vi "Measurement_input_panel.vi"(0 "OK":T4, 2 "setup":T5, 5 "Setup filename":string) -> (11 "Setup filename out":string, 12 "Analysis Info cluster":T8[](array[typedef])=[{"Colour"=0, "Inst type"=enum."Pitot-static tube", "Inst name"="Manometer voltage", "Symbol"="U", "Code name"="", "Extra Info"="U", "Inst Array"=enum."PWA", "Extra Titles"=[], "Extra Values"=[], "U"=0.0, "u^2"=0.0, "u^3"=0.0, "u^4"=0.0, "Skew_u"=0.0, "Kurt_u"=0.0, "Sd Error in Mean"=0.0, "% u'/U"=0.0, "X"=0.0, "Y"=0.0, "Z"=0.0, "Timescale integral to 25%"=0.0, "Sd Error in Variance"=0.0, "Calib File"=path "", "Calib Constants"=[], "Output Position"=FALSE, "Full Stats"=FALSE, "Av Sampling Rate"=0.0, "Av No of Samples"=0.0, "Total Meas Time (s)"=0.0, "ADAM Ch Name"=""}, {"Colour"=0, "Inst type"=enum."Pitot-static tube", "Inst name"="Manometer voltage", "Symbol"="U", "Code name"="", "Extra Info"="U", "Inst Array"=enum."PWA", "Extra Titles"=[], "Extra Values"=[], "U"=0.0, "u^2"=0.0, "u^3"=0.0, "u^4"=0.0, "Skew_u"=0.0, "Kurt_u"=0.0, "Sd Error in Mean"=0.0, "% u'/U"=0.0, "X"=0.0, "Y"=0.0, "Z"=0.0, "Timescale integral to 25%"=0.0, "Sd Error in Variance"=0.0, "Calib File"=path "", "Calib Constants"=[], "Output Position"=FALSE, "Full Stats"=FALSE, "Av Sampling Rate"=0.0, "Av No of Samples"=0.0, "Total Meas Time (s)"=0.0, "ADAM Ch Name"=""}, {"Colour"=0, "Inst type"=enum."Pitot-static tube", "Inst name"="Manometer voltage", "Symbol"="U", "Code name"="", "Extra Info"="U", "Inst Array"=enum."PWA", "Extra Titles"=[], "Extra Values"=[], "U"=0.0, "u^2"=0.0, "u^3"=0.0, "u^4"=0.0, "Skew_u"=0.0, "Kurt_u"=0.0, "Sd Error in Mean"=0.0, "% u'/U"=0.0, "X"=0.0, "Y"=0.0, "Z"=0.0, "Timescale integral to 25%"=0.0, "Sd Error in Variance"=0.0, "Calib File"=path "", "Calib Constants"=[], "Output Position"=FALSE, "Full Stats"=FALSE, "Av Sampling Rate"=0.0, "Av No of Samples"=0.0, "Total Meas Time (s)"=0.0, "ADAM Ch Name"=""}] {"Sd Error in Variance" format="%.2f"; "Skew_u" format="%.2f"; "% u'/U" format="%.2f"; "Sd Error in Mean" format="%.2f"; "Kurt_u" format="%.2f"; "u^4" format="%.2f"; "u^3" format="%.2f"; "U" format="%.2f"; "u^2" format="%.2f"})   [LabVIEW 2012]
uses:
  Controls/Inst_type.ctl
  Controls/Analysis_info_cluster.ctl
  Controls/Instrument_Array.ctl
  Controls/LDA_Setup.ctl
  Controls/Setup.ctl
  Controls/ok_button.ctl
  Controls/Trigger_Mode.ctl
  Controls/PWA_Data.ctl
  File/Setup_Filetype.ctl
  Controls/Post_Process.ctl
  Controls/App_Global.ctl
  Controls/Ch_and_Spans.ctl
  Globals/Meas_global.vi
  Globals/Trav_pos_global.vi
  Globals/LDA_meas_global_1.vi
  Globals/Preference_global.vi
panel:
  in  "Acquisition Plug in":u16(ring) items=["ADAM_Server_Channels.vi", "DataTranslation.vi", "DataTranslation_new.vi", "DataTranslation_NM1.vi", "DataTranslation_NM2.vi", "DataTranslation_NM3.vi", "DataTranslation_old.vi", "LDA_IP.vi", "LDA_IP_DataTranslation.vi", "LDA_IP_NI-DAQmx.vi", "NI-DAQmx.vi", "Simulate_kernal.vi"]
  in  "Select Duplicate Channels":bool
  in  "PWA Data":T1
  out "Inst type":T2
  in  "Edit temp and Press":bool
  out "Abs Press (mbar)":dbl=1013.0 format="%.1f"
  out "Temp (deg C)":dbl=21.0 format="%.1f"
  in  "Trigger mode":T3
  in  "Select Plug Ins":bool
  in  "Sync Delay Time (ms)":dbl=24.0 format="%.2f"
  out "XW Present?":bool
  out "Read Setup File?":bool
  out "Setup Paths":string[](array[string])
  in  "Select Local ADAM Channels":bool
  in  "stop":bool
  out "Notes":string
  in  "Setup filename selector":u16(ring) items=["Current_Setup.xls", "Disp_Search_A.xls", "Calib_Setup.xls", "Simulate.xls", "LDA_SJ_A.xls", "LDA_only_B.xls", "LDA_only_A.xls", "NACA0015_Pressure_LDA.xls", "NACA0015_Pressure.xls", "Current_Setup.xls", "NACA0015_Pressure_LDA.xls", "NACA0015_Pressure.xls", "DT9836_test.xls", "DT_test_C.xls", "LDA_Test.xls", "SJ_Span_Test_B.xls", "DT_test_B.xls", "DT_test.xls", "NACA0015_SJ_Polar_B.xls", "NACA0015_RT_Pres_A.xls", "NACA0015_SJ_Polar_A.xls", "Calib_Setup.xls", "SJ_Indv_Test_B.xls", "NACA0015_RT_Pres_B.xls", "NACA0015_LDA_A.xls", "SJ_Indv_Test_A.xls", "SJ_Span_Test_A.xls", "NACA0015_Polar_C.xls", "SJ_Disp_A.xls", "LDA_C.xls", "SJ_Life_Test_A.xls", "LDA_D.xls", "Tare_Setup.xls", "NACA0015_Polar_B.xls", "LDA_B.xls", "LDA_A.xls", "NACA0015_Polar_A.xls", "Meas_Test.xls", "SJ_Optimisation_A.xls", "Fluidic_Switch_B.xls", "SJ_Test_Alex_A.xls", "Fluidic_Switch_A.xls", "SJ_Steel_Rig_C.xls", "SJ_Steel_Rig_B.xls", "SJ_Steel_Rig_A.xls", "HW_Calibrate_A.xls"]
  in  "Synchronise Analogue channels with LDA":bool
  in  "LDA set up":T6={"dimensions"=enum."2D", "Analogue Freq Multiplier"=0.1} {"Analogue Freq Multiplier" min=0.1 max=100.0 format="%_5g"}
  in  "LDA data":enum16{"No LDA data", "Take LDA data"}(ring)=enum."Take LDA data"
  in  "Cross wire":T7(ring)
  in  "No of Analogue inst":i32=1
  in  "Ch & spans choices":T10(array[cluster]) {"D" format="%.2f"; "Ch No" min=0; "low limit" min=-10 max=10 format="%.2f"; "high limit" min=-10 max=10 format="%.2f"}
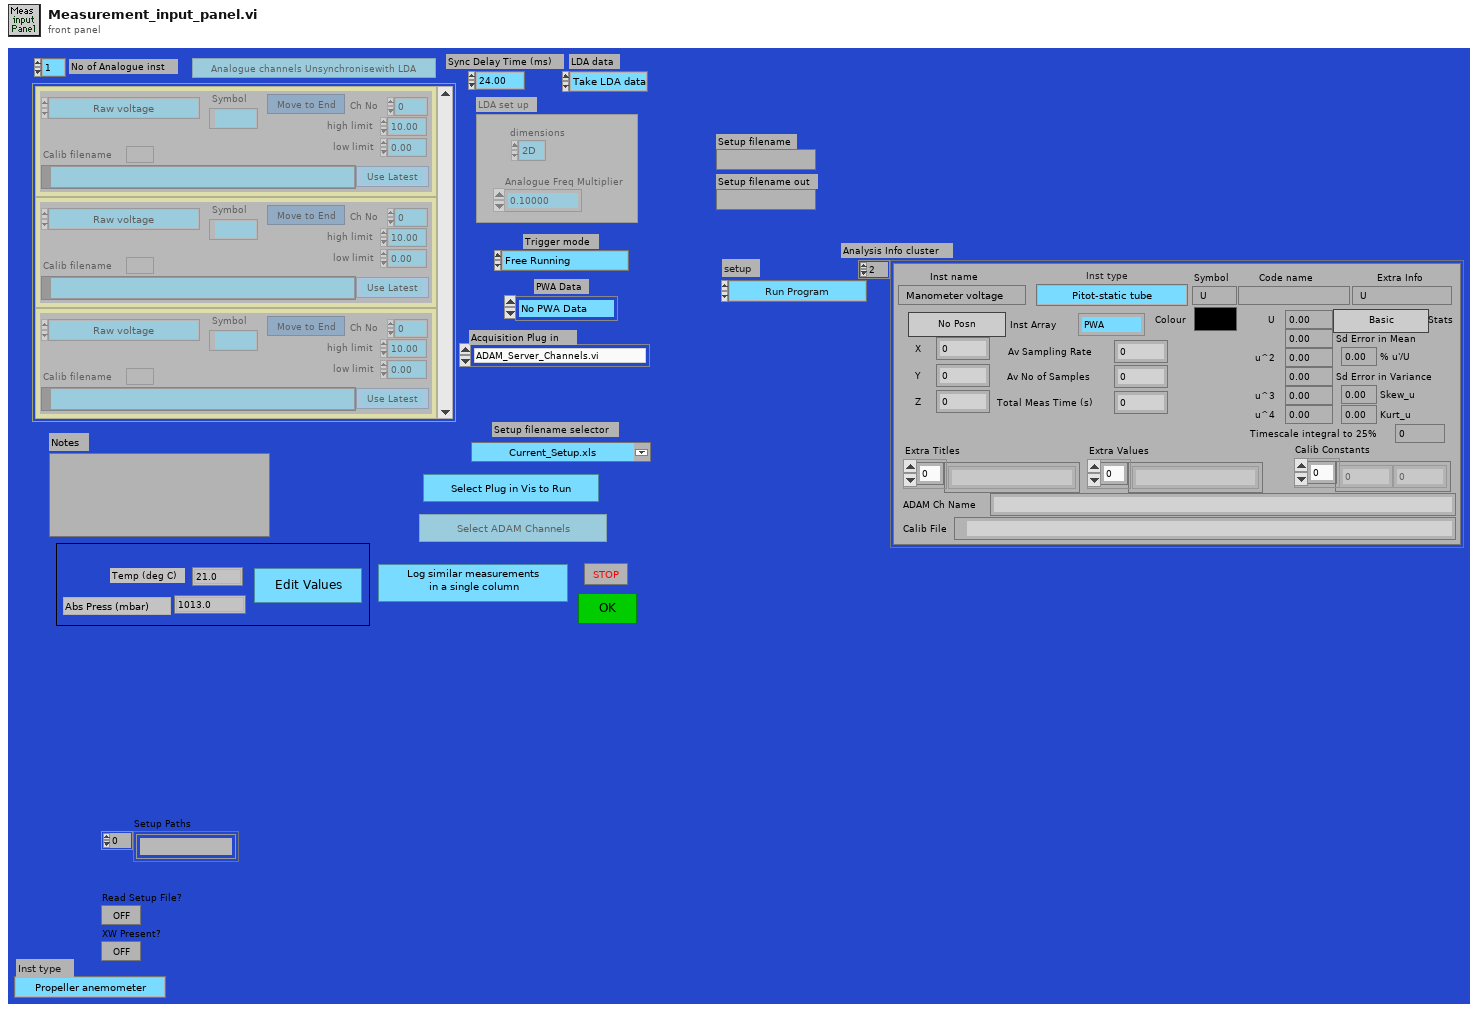
[diagram p1: front panel]
types:
  T1 = typedef "PWA_Data.ctl" = enum16{"No PWA Data", "One Ch PWA"}
  T2 = typedef "Inst_type.ctl" = enum16{"Propeller anemometer", "Raw voltage", "Pressure Transducer", "Pitot-static tube", "Preston tube", "Hot wire", "Cross wire 1", "Cross wire 2", "Generic Linear", "Generic Polynomial", "Generic BackPoly", "Fast FID", "Thermocouple", "Cold wire", "Pulsed Wire", "LDA Vel", "LDA Tran time", "LDA Arr time"}
  T3 = typedef "Trigger_Mode.ctl" = enum16{"Free Running", "Start on Trigger", "Trigger Every Block", "Trigger Every Sample"}
  T4 = typedef "ok_button.ctl" = bool
  T5 = typedef "Setup.ctl" = enum16{"Run Program", "Show Setup", "Save Current Setup", "Setup Front Panel"}
  T6 = typedef "LDA_Setup.ctl" = cluster{"dimensions":enum16{"1D", "2D"}, "Analogue Freq Multiplier":dbl}
  T7 = enum16{"2nd component as calculated", "2nd component multipled by -1"}
  T8 = typedef "Analysis_info_cluster.ctl" = cluster{"Colour":u32, "Inst type":T2, "Inst name":string, "Symbol":string, "Code name":string, "Extra Info":string, "Inst Array":T9, "Extra Titles":string[], "Extra Values":string[], "U":dbl, "u^2":dbl, "u^3":dbl, "u^4":dbl, "Skew_u":dbl, "Kurt_u":dbl, "Sd Error in Mean":dbl, "% u'/U":dbl, "X":dbl, "Y":dbl, "Z":dbl, "Timescale integral to 25%":dbl, "Sd Error in Variance":dbl, "Calib File":path, "Calib Constants":dbl[], "Output Position":bool, "Full Stats":bool, "Av Sampling Rate":dbl, "Av No of Samples":dbl, "Total Meas Time (s)":dbl, "ADAM Ch Name":string}
  T9 = typedef "Instrument_Array.ctl" = enum16{"PWA", "LDA", "Analogue"}
  T10 = cluster{"high limit":sgl, "low limit":sgl, "Ch No":i16, "Calib filename":path, "Inst type":T2, "Symbol":string, "Move channel":bool, "Use Latest":bool, "D":dbl, "Ch Name":string}[]
  T11 = typedef "Post_Process.ctl" = enum16{"Take New Data", "Post Process Raw Data File"}
  T12 = typedef "Setup_Filetype.ctl" = enum16{"Measurement Setups", "Calibration Setups", "General", "Results File Plotter Setups", "Speed Calib Tweaks"}
  T13 = typedef "App_Global.ctl" = enum16{"Read Global", "Write to Global", "Initialise Array"}
  T14 = typedef "Ch_and_Spans.ctl" = cluster{"high limit (10V)":sgl, "low limit (-10V)":sgl, "Ch No":i16, "Var name":string, "Use Latest Calib":bool}
  T15 = enum16{"Zero or one", "One", "Zero or more", "One or more"}
  T16 = typedef "Traverse_cluster.ctl" = cluster{"Start X":dbl, "Start Y":dbl, "Start Z":dbl, "End X":dbl, "End Y":dbl, "End Z":dbl, "No. of pts.":i32, "Spacing":T17, "Filename":path, "Tunnel Speed":dbl, "Averaging time (min)":dbl, "Extra Commands":string, "Specific Arguments":string, "Emission Rate (l/min)":dbl, "Trace Gas Concentration (%)":dbl, "Density Ratio":string, "Comments":string, "Row No":i32, "Row Type Selector":T18, "Completion time":string, "Row Duration (mins)":dbl, "No. of Valid pts.":i32, "Meas Setup File":string}
  T17 = typedef "Spacing.ctl" = enum16{"Linear", "Log", "Gauss", "Specified", "N/A"}
  T18 = typedef "Multi_run_mode.ctl" = enum16{"Move Traverse Only", "Set Tunnel Speed Only", "Set Source Only", "Set Measurement Conditions", "Single Measurement", "Vertical Profile", "Lateral Profile", "Longitudinal Profile", "Explore Volume", "Multi-Axis Profile", "Auto Calibrate", "Meas Fast FID Bkgnd", "Check Beam Power", "Scanning Valve Measurement", "Run VI Named:", "Set ADAM Ch", "Wait (minutes)", "Send Message", "Synchronize With:", "Fall Back to this Row", "Turn Off Row Repeating", "Blank Row", "Traverse 3D Volume"}
  T19 = cluster{"high limit (10V)":sgl, "low limit (-10V)":sgl, "Ch No":i16, "Calib filename":path, "Inst type":T2, "Symbol":string, "Move channel":bool, "Use Latest":bool, "D":dbl, "Ch Name":string}[]
  T20 = cluster{"high limit":sgl, "low limit":sgl, "Ch No":i16, "Calib filename":path, "Inst type":T2, "Symbol":string, "Move channel":bool, "Use Latest":bool, "D":dbl, "Ch Name":string}
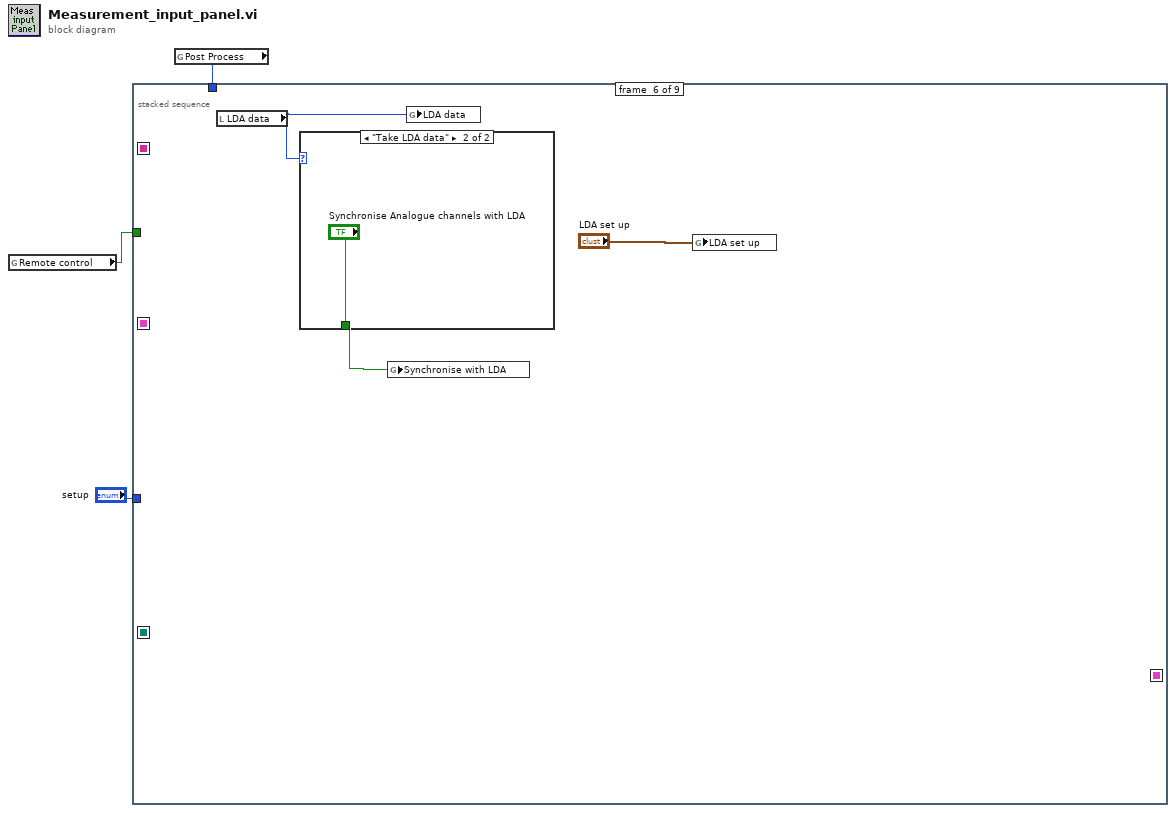
[diagram p0: block diagram]
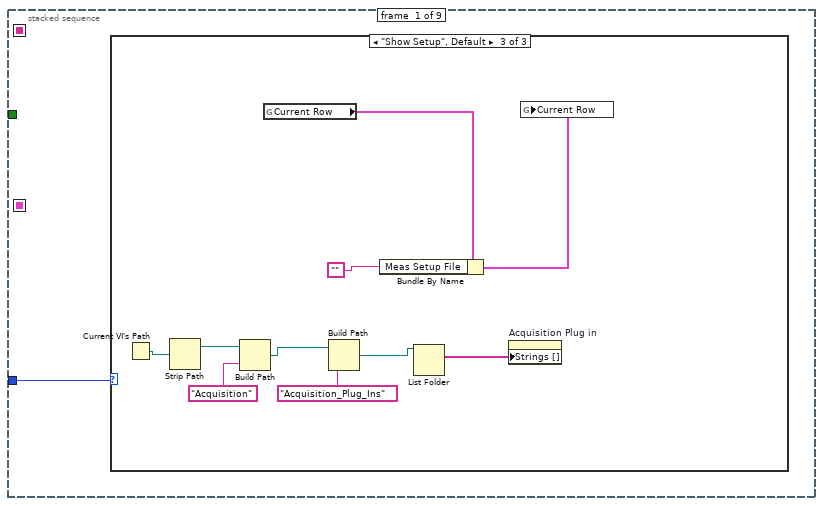
[diagram p2: hidden frame]
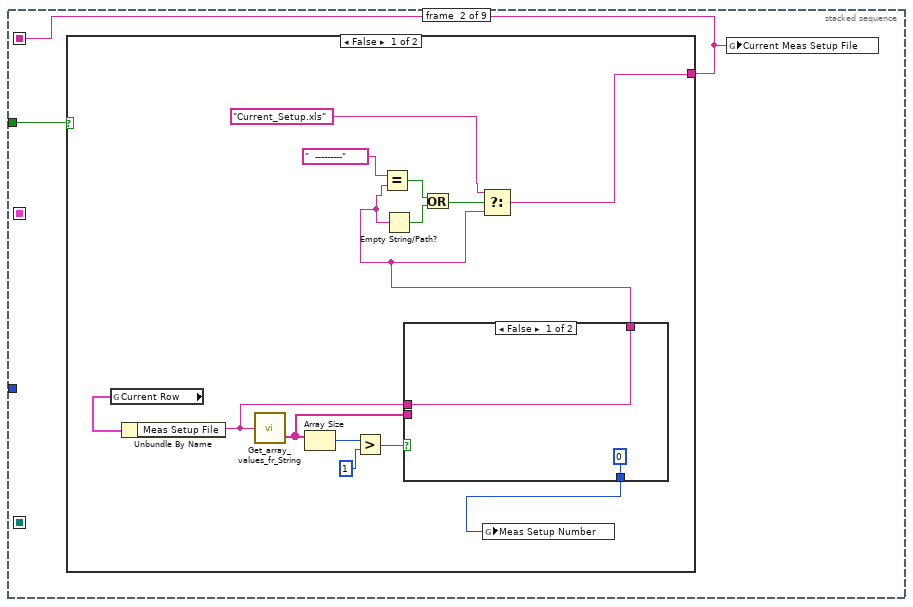
[diagram p5: hidden frame]
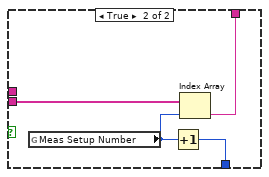
[diagram p6: hidden frame]
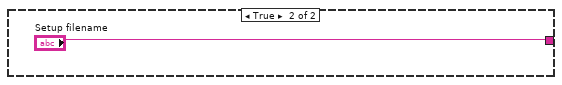
[diagram p7: hidden frame]
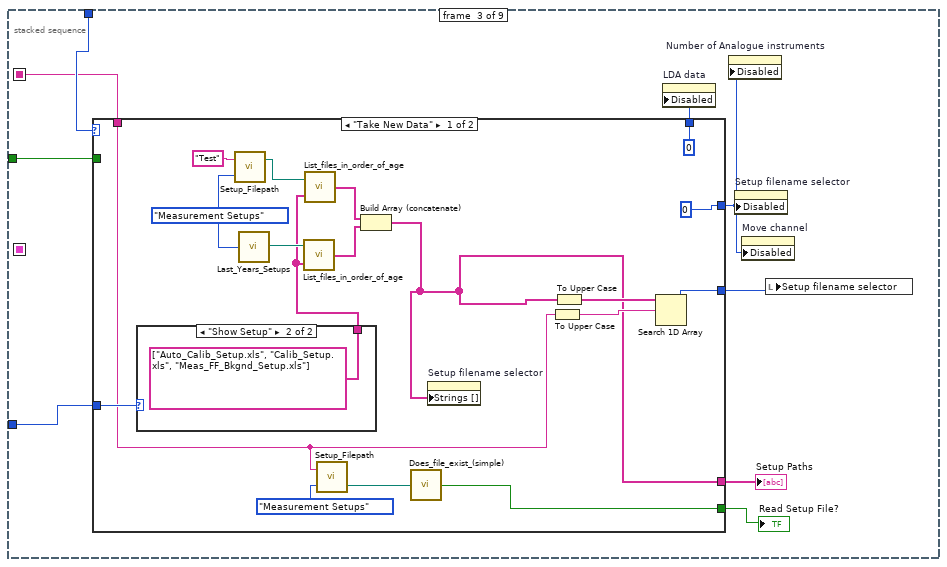
[diagram p8: hidden frame]
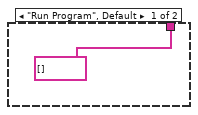
[diagram p9: hidden frame]
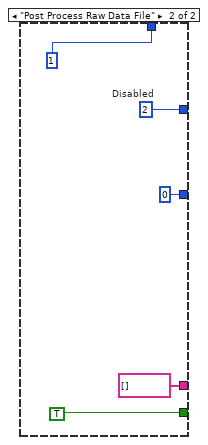
[diagram p10: hidden frame]
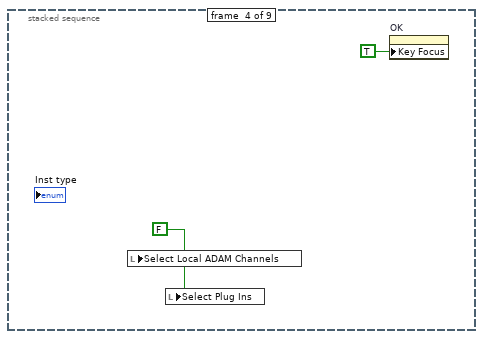
[diagram p11: hidden frame]
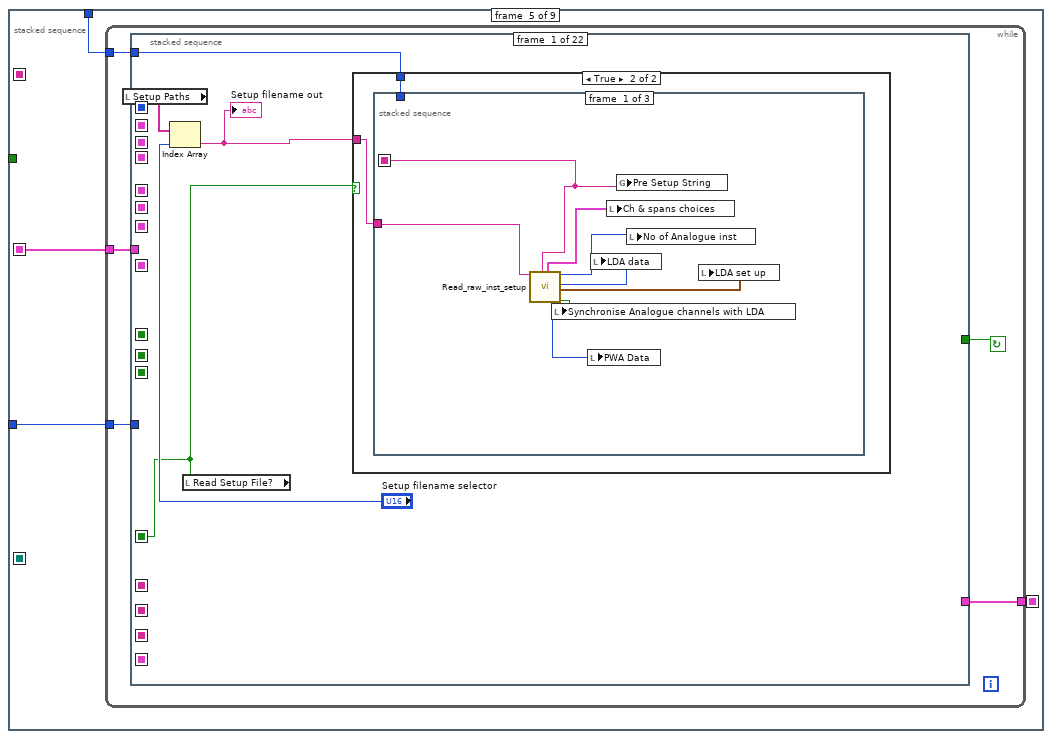
[diagram p12: hidden frame]
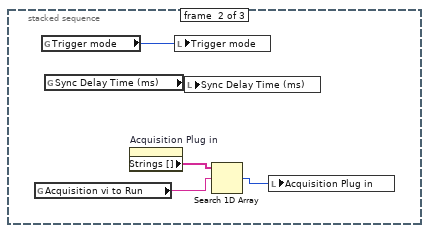
[diagram p14: hidden frame]
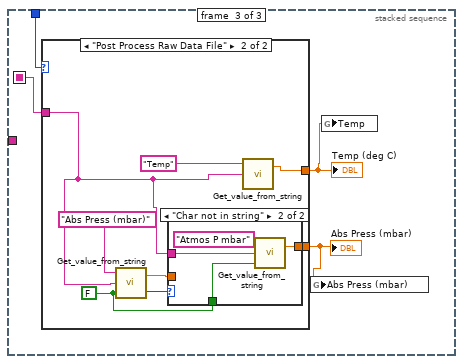
[diagram p15: hidden frame]
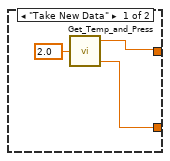
[diagram p16: hidden frame]
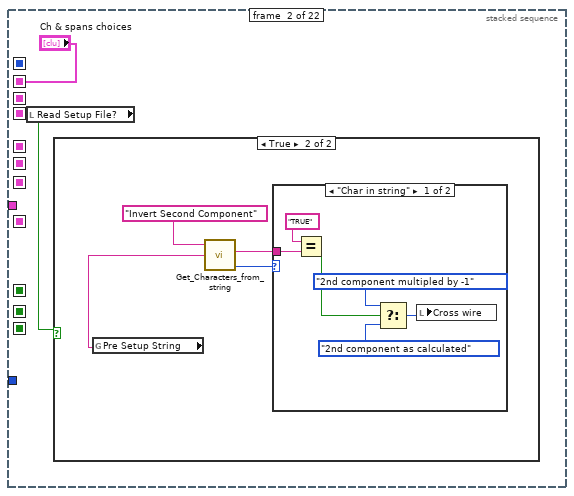
[diagram p18: hidden frame]
diagram:
  n1 = global read "Meas_global.vi" "Remote control"() -> (w1:bool)
  n2 = global read "Meas_global.vi" "Post Process"() -> (w3:T11)
  n3 = stacked-sequence {
    seq-local: [_ _ _ _ w77 _ _ _ _] -> [_ _ _ _ _ _ w693 w794 _]
    seq-local: [_ w15 _ _ _ _ _ _ _] -> [_ _ w38 _ _ _ w692 _ _]
    seq-local: [_ _ _ _ w74 _ _ _ _] -> [_ _ _ _ _ _ _ _ w846]
    seq-local: [_ _ _ _ _ _ _ w793 _] -> [_ _ _ _ _ _ _ _ w845]
    tunnel: w3 -> [_ _ w46 _ w76 _ _ w795 _]
    tunnel: "setup" -> [w4 _ w40 _ w75 _ w694 _ _]
    tunnel: w1 -> [_ w16 w39 _ _ _ _ _ _]
    frame #0 {
      n4 = case shown="\"Show Setup\", Default" w4 {
        frame "Run Program" {
        }
        frame "Setup Front Panel" {
        }
        frame "Show Setup", Default {
          n5 = Current VI's Path() -> (path=w11:path)
          n6 = Strip Path(path=w11) -> (stripped path=w10:path)  [unwired: 1 out]
          n7 = Build Path(base path=w10, name or relative path="Acquisition") -> (appended path=w7:path)
          n8 = global read "Trav_pos_global.vi" "Current Row"() -> (w14:T16)
          n9 = Build Path(base path=w7, name or relative path="Acquisition_Plug_Ins") -> (appended path=w6:path)
          n10 = Bundle By Name(cluster=w14, "Meas Setup File"="") -> (w13:T16)
          n11 = List Folder(path=w6) -> (filenames=w5:string[])  [unwired: 3 in, 3 out]
          n12 = property on="Acquisition Plug in" class="Ring (strict)"("Strings []"=w5) -> ()  [unwired: 2 in, 2 out]
          n13 = global write "Trav_pos_global.vi" "Current Row"(w13) -> ()
        }
      }
    }
    frame #1 {
      n14 = case shown="False" w16 {
        tunnel: [w29 "Setup filename"] -> w15
        frame False {
          n15 = global read "Trav_pos_global.vi" "Current Row"() -> (w25:T16)
          n16 = Unbundle By Name(w25) -> ("Meas Setup File"=w19:string)
          n17 = call "Get_array_values_fr_String.vi"("String Value"=w19) -> ("String array"=w18:string[])  [unwired: 1 out]
          n18 = Array Size(array=w18) -> (size(s)=w23:i32)
          n19 = Greater?(x=w23, y=1) -> (0:w21:bool)
          n20 = case shown="False" w21 {
            tunnel: [w32 w35] -> w20
            tunnel: w19 -> [w32 _]
            tunnel: w18 -> [_ w36]
            tunnel: [0 w33] -> w17
            frame False {
            }
            frame True {
              n21 = global read "Trav_pos_global.vi" "Meas Setup Number"() -> (w34:i32)
              n22 = Increment(x=w34) -> (x+1=w33:i32)
              n23 = Index Array(array=w36, index=w34) -> (element=w35:string)
            }
          }
          n24 = Equal?(x="  ---------" ("f"), y=w20) -> (x = y?=w28:bool)
          n25 = Empty String/Path?(string/path=w20) -> (empty?=w27:bool)
          n26 = Or(x=w28, y=w27) -> (x .or. y?=w24:bool)
          n27 = Select(t="Current_Setup.xls", s=w24, f=w20) -> (s? t:f=w29:string)
          n28 = global write "Trav_pos_global.vi" "Meas Setup Number"(w17) -> ()
        }
        frame True {
        }
      }
      n29 = global write "Trav_pos_global.vi" "Current Meas Setup File"(w15) -> ()
    }
    frame #2 {
      n30 = case shown="\"Take New Data\"" w46 {
        tunnel: [w47 string[] []] -> w42
        tunnel: [w60 TRUE ("exists")] -> w41
        tunnel: [u8 0 ("Disabled") w68] -> w43
        tunnel: [u8 0 ("Disabled") u8 1 ("Disabled")] -> w45
        tunnel: w38 -> [w56 _]
        tunnel: [w63 0 ("index of element")] -> w44
        tunnel: w40 -> [w58 _]
        tunnel: w39 -> [_ _]
        frame "Take New Data" {
          w50 = Setup_Filetype."Measurement Setups" ("Setup File Type")
          n31 = case shown="\"Show Setup\"" w58 {
            tunnel: [string[] [] ("file names") string[] ["Auto_Calib_Setup.xls", "Calib_Setup.xls", "Meas_FF_Bkgnd_Setup.xls"] ("file names")] -> w48
            frame "Run Program", Default {
            }
            frame "Show Setup" {
            }
          }
          n32 = call "Setup_Filepath.vi"("Setup File Type"=w50, "Filename in"="Test") -> ("Directory"=w51:path)  [unwired: 1 out]
          n33 = call "Last_Years_Setups.vi"("Setup File Type"=w50) -> ("Directory"=w49:path)
          n34 = call "List_files_in_order_of_age.vi"("Files to Hide"=w48, "Folder"=w49) -> ("file names"=w53:string[])
          n35 = call "List_files_in_order_of_age.vi"("Files to Hide"=w48, "Folder"=w51) -> ("file names"=w52:string[])
          n36 = call "Setup_Filepath.vi"("Setup File Type"=Setup_Filetype."Measurement Setups", "Filename in"=w56) -> ("Filename Out"=w55:path)  [unwired: 1 out]
          n37 = Build Array (concatenate)(w52, w53) -> (w47:string[])
          n38 = call "Does_file_exist_(simple).vi"("Pathname"=w55) -> ("exists?"=w60:bool)
          n39 = property on="Setup filename selector" class="Ring (strict)"("Strings []"=w47) -> ()  [unwired: 2 in, 2 out]
          n40 = To Upper Case(1:w56) -> (0:w61:string)
          n41 = To Upper Case(1:w47) -> (0:w62:string[])
          n42 = Search 1D Array(1D array=w62, element=w61) -> (index of element=w63:i32)  [unwired: 1 out]
        }
        frame "Post Process Raw Data File" {
          w68 = u8 2  # Disabled
        }
      }
      "Setup Paths" <- w42
      "Read Setup File?" <- w41
      n43 = property on="LDA data" class="Enum (strict)"("Disabled"=w45) -> ()  [unwired: 2 in, 2 out]
      n44 = property on="Number of Analogue instruments" class="DigNum (strict)"("Disabled"=w43) -> ()  [unwired: 2 in, 2 out]
      n45 = property on="Setup filename selector" class="Ring (strict)"("Disabled"=w43) -> ()  [unwired: 2 in, 2 out]
      n46 = property on="Move channel" class="Bool (strict)"("Disabled"=w43) -> ()  [unwired: 2 in, 2 out]
      n47 = local write "Setup filename selector"(w44) -> ()
    }
    frame #3 {
      w73 = FALSE ("Select Local ADAM Channels")
      n48 = local write "Select Local ADAM Channels"(w73) -> ()
      n49 = local write "Select Plug Ins"(w73) -> ()
      n50 = property on="OK" class="Bool"("Key Focus"=TRUE) -> ()  [unwired: 2 in, 2 out]
    }
    frame #4 {
      n51 = while {
        tunnel: w75 -> [w79]
        tunnel: w76 -> [w80]
        tunnel: [w82] -> w77
        tunnel: [w78] -> w74
        stop <- w81 continue-if-true
        n52 = stacked-sequence {
          seq-local: [_ _ _ _ _ _ _ _ _ w238 _ _ _ _ _ _ _ _ _ _ _ _] -> [_ _ _ _ _ _ _ _ _ _ _ w301 w346 w391 _ _ _ _ _ _ _ _]
          seq-local: [_ _ _ _ w162 _ _ _ _ _ _ _ _ _ _ _ _ _ _ _ _ _] -> [_ _ _ _ _ _ w200 _ w234 w239 _ _ _ _ _ _ _ _ _ _ _ _]
          seq-local: [_ _ _ _ _ _ w205 _ _ _ _ _ _ _ _ _ _ _ _ _ _ _] -> [_ _ _ _ _ _ _ _ _ w240 _ _ _ _ _ _ _ _ _ _ _ _]
          seq-local: [_ _ _ _ _ _ _ _ _ _ _ w303 _ _ _ _ _ _ _ _ _ _] -> [_ _ _ _ _ _ _ _ _ _ _ _ w348 _ _ _ _ _ _ _ _ w658]
          seq-local: [_ _ _ _ _ _ _ _ _ _ _ _ _ _ w424 _ _ _ _ _ _ _] -> [_ _ _ _ _ _ _ _ _ _ _ _ _ _ _ w443 _ _ _ _ _ _]
          seq-local: [_ _ _ _ _ _ _ _ _ _ _ _ _ _ _ w439 _ _ _ _ _ _] -> [_ _ _ _ _ _ _ _ _ _ _ _ _ _ _ _ w467 w533 _ _ w634 w659]
          seq-local: [_ _ _ _ _ _ _ _ _ _ _ _ w352 _ _ _ _ _ _ _ _ _] -> [_ _ _ _ _ _ _ _ _ _ _ _ _ _ w421 _ _ _ _ _ _ _]
          seq-local: [_ _ _ _ _ _ _ _ _ _ _ _ _ w395 _ _ _ _ _ _ _ _] -> [_ _ _ _ _ _ _ _ _ _ _ _ _ _ w420 _ _ _ _ _ _ _]
          seq-local: [_ _ _ _ _ _ _ _ _ _ w298 _ _ _ _ _ _ _ _ _ _ _] -> [_ _ _ _ _ _ _ _ _ _ _ w302 w349 _ _ _ _ _ _ _ _ w657]
          seq-local: [_ _ _ _ _ _ _ _ _ _ _ _ _ _ _ _ w466 _ _ _ _ _] -> [_ _ _ _ _ _ _ _ _ _ _ _ _ _ _ _ _ w536 _ _ _ _]
          seq-local: [_ _ _ _ _ _ _ _ _ _ _ _ _ _ _ _ w465 _ _ _ _ _] -> [_ _ _ _ _ _ _ _ _ _ _ _ _ _ _ _ _ w535 _ _ _ _]
          seq-local: [_ _ _ _ _ _ _ _ _ _ _ _ _ _ _ _ w464 _ _ _ _ _] -> [_ _ _ _ _ _ _ _ _ _ _ _ _ _ _ _ _ w534 _ _ _ _]
          seq-local: [_ _ _ _ _ _ _ _ _ _ _ _ _ _ _ _ _ w532 _ _ _ _] -> [_ _ _ _ _ _ _ _ _ _ _ _ _ _ _ _ _ _ _ w584 _ _]
          seq-local: [_ "Ch & spans choices" _ _ _ _ _ _ _ _ _ _ _ _ _ _ _ _ _ _ _ _] -> [_ _ _ _ w151 _ _ _ _ _ _ _ _ _ _ _ _ _ w579 _ _ _]
          seq-local: [_ _ _ _ _ _ _ _ _ _ _ _ _ _ _ _ _ w530 _ _ _ _] -> [_ _ _ _ _ _ _ _ _ _ _ _ _ _ _ _ _ _ w578 _ _ _]
          seq-local: [w83 _ _ _ _ _ _ _ _ _ _ _ _ _ _ _ _ _ _ _ _ _] -> [_ _ _ _ _ _ _ _ _ _ _ _ _ _ _ _ _ w529 _ _ _ _]
          tunnel: [_ _ _ _ _ _ _ _ _ _ _ _ _ _ _ w439 _ _ _ _ _ _] -> w82
          tunnel: [_ _ _ _ _ _ _ _ _ _ _ _ w350 _ _ _ _ _ _ _ _ _] -> w81
          tunnel: w80 -> [w85 _ _ w139 w158 _ _ _ _ _ w299 _ w347 _ w423 _ _ _ _ _ w635 _]
          tunnel: w79 -> [_ _ w135 _ _ w186 _ _ _ _ _ _ _ _ w422 _ _ _ _ w586 _ _]
          tunnel: [_ _ _ _ _ _ _ _ _ _ _ _ _ _ _ _ _ w532 _ _ _ _] -> w78
          frame #0 {
            n53 = local read "Setup Paths"() -> (w87:string[])
            n54 = Index Array(array=w87, index="Setup filename selector") -> (element=w84:string)
            "Setup filename out" <- w84
            n55 = local read "Read Setup File?"() -> (w83:bool)
            n56 = case shown="True" w83 {
              tunnel: w84 -> [_ w89]
              tunnel: w85 -> [_ w88]
              frame False {
              }
              frame True {
                n57 = stacked-sequence {
                  seq-local: [w92 _ _] -> [_ _ w105]
                  tunnel: w89 -> [w94 _ _]
                  tunnel: w88 -> [_ _ w106]
                  frame #0 {
                    n58 = call "Read_raw_inst_setup.vi"("Setup file"=w94) -> ("Setup string"=w92:string, "Ch & spans choices"=w91:T19, "PWA Data"=w90:T1, "Number of Analogue instruments"=w97:i32, "LDA data"=w96:enum16{"No LDA data", "Take LDA data"}, "LDA set up"=w93:T6, "Synchronise Analogue channels with LDA"=w95:bool)  [unwired: 12 out]
                    n59 = local write "Synchronise Analogue channels with LDA"(w95) -> ()
                    n60 = local write "PWA Data"(w90) -> ()
                    n61 = local write "LDA data"(w96) -> ()
                    n62 = local write "Ch & spans choices"(w91) -> ()
                    n63 = global write "Meas_global.vi" "Pre Setup String"(w92) -> ()
                    n64 = local write "No of Analogue inst"(w97) -> ()
                    n65 = local write "LDA set up"(w93) -> ()
                  }
                  frame #1 {
                    n66 = global read "Meas_global.vi" "Acquisition vi to Run"() -> (w99:string)
                    n67 = global read "Meas_global.vi" "Trigger mode"() -> (w101:T3)
                    n68 = global read "LDA_meas_global_1.vi" "Sync Delay Time (ms)"() -> (w102:dbl)
                    n69 = property on="Acquisition Plug in" class="Ring (strict)"() -> ("Strings []"=w100:string[])  [unwired: 2 in, 2 out]
                    n70 = local write "Trigger mode"(w101) -> ()
                    n71 = local write "Sync Delay Time (ms)"(w102) -> ()
                    n72 = Search 1D Array(1D array=w100, element=w99) -> (index of element=w98:i32)  [unwired: 1 in]
                    n73 = local write "Acquisition Plug in"(w98) -> ()
                  }
                  frame #2 {
                    n74 = case shown="\"Post Process Raw Data File\"" w106 {
                      tunnel: w105 -> [_ w112]
                      tunnel: [w107 w111] -> w103
                      tunnel: [w108 w110] -> w104
                      frame "Take New Data" {
                        n75 = call "Get_Temp_and_Press.vi"("Averaging time (mins)"=2.0) -> ("Abs Press (mbar)"=w107:dbl, "Temperature"=w108:dbl)  [unwired: 3 out]
                      }
                      frame "Post Process Raw Data File" {
                        w114 = FALSE ("Show Dialog?")
                        n76 = call "Get_value_from_string.vi"("Show Dialog?"=w114, "Input string"=w112, "Variable name"="Abs Press (mbar)") -> ("Status"=w116:enum16{"Char in string", "Char not in string"}, "Value"=w115:dbl)
                        n77 = case shown="\"Char not in string\"" w116 {
                          tunnel: [w118 w121] -> w111
                          tunnel: w115 -> [w118 _]
                          tunnel: w114 -> [_ w120]
                          tunnel: w112 -> [_ w119]
                          frame "Char in string" {
                          }
                          frame "Char not in string" {
                            n78 = call "Get_value_from_string.vi"("Show Dialog?"=w120, "Input string"=w119, "Variable name"="Atmos P mbar") -> ("Value"=w121:dbl)  [unwired: 1 out]
                          }
                        }
                        n79 = call "Get_value_from_string.vi"("Input string"=w112, "Variable name"="Temp") -> ("Value"=w110:dbl)  [unwired: 1 in, 1 out]
                      }
                    }
                    "Abs Press (mbar)" <- w103
                    "Temp (deg C)" <- w104
                    n80 = global write "Meas_global.vi" "Abs Press (mbar)"(w103) -> ()
                    n81 = global write "Meas_global.vi" "Temp"(w104) -> ()
                  }
                }
              }
            }
          }
          frame #1 {
            n82 = local read "Read Setup File?"() -> (w124:bool)
            n83 = case shown="True" w124 {
              frame False {
              }
              frame True {
                n84 = global read "Meas_global.vi" "Pre Setup String"() -> (w127:string)
                n85 = call "Get_Characters_from_string.vi"("Input string"=w127, "Variable name"="Invert Second Component") -> ("Status"=w126:enum16{"Char in string", "Char not in string"}, "Value"=w125:string)  [unwired: 1 in]
                n86 = case shown="\"Char in string\"" w126 {
                  tunnel: w125 -> [w134 _]
                  frame "Char in string" {
                    n87 = Equal?(x="TRUE", y=w134) -> (x = y?=w130:bool)
                    n88 = Select(t=T7."2nd component multipled by -1" ("Cross wire/LDA"), s=w130, f=T7."2nd component as calculated" ("Cross wire/LDA")) -> (s? t:f=w132:T7)
                    n89 = local write "Cross wire"(w132) -> ()
                  }
                  frame "Char not in string" {
                  }
                }
              }
            }
          }
          frame #2 {
            n90 = case shown="\"Show Setup\"" w135 {
              frame "Run Program", Default {
              }
              frame "Show Setup" {
                n91 = property on="Acquisition Plug in" class="Ring (strict)"() -> ("Strings []"=w138:string[])  [unwired: 2 in, 2 out]
                n92 = Index Array(array=w138, index="Acquisition Plug in") -> (element=w136:string)
                n93 = global write "Meas_global.vi" "Acquisition vi to Run"(w136) -> ()
              }
            }
          }
          frame #3 {
            n94 = case shown="True" "Edit temp and Press" {
              tunnel: w139 -> [_ w141]
              frame False {
              }
              frame True {
                n95 = case shown="\"Take New Data\"" w141 {
                  frame "Take New Data" {
                    n96 = stacked-sequence {
                      frame #0 {
                        w142 = TRUE  # Wait until done
                        n97 = call "Run_Enter_Temp.vi"("Wait until done"=w142) -> ()  [unwired: 1 out]
                      }
                      frame #1 {
                        n98 = call "Get_Temp_and_Press.vi"("Averaging time (mins)"=2.0) -> ("Abs Press (mbar)"=w143:dbl, "Temperature"=w144:dbl)  [unwired: 3 out]
                        n99 = local write "Temp (deg C)"(w144) -> ()
                        n100 = local write "Abs Press (mbar)"(w143) -> ()
                      }
                    }
                  }
                  frame "Post Process Raw Data File" {
                  }
                }
              }
            }
          }
          frame #4 {
            w154 = u8 0  # Disabled
            n101 = local read "Read Setup File?"() -> (w150:bool)
            n102 = global read "Meas_global.vi" "Acquisition vi to Run"() -> (w149:string)
            n103 = Equal?(x=w158, y=Post_Process."Take New Data" ("Post Process")) -> (x = y?=w157:bool)
            n104 = Equal?(x="ADAM_Server_Channels.vi", y=w149) -> (x = y?=w147:bool)
            n105 = And(x=w150, y=w147) -> (x .and. y?=w161:bool)
            n106 = Or(x="Select Local ADAM Channels", y=w161) -> (x .or. y?=w155:bool)
            n107 = And(x=w157, y=w155) -> (x .and. y?=w156:bool)
            n108 = case shown="True" w156 {
              tunnel: [w163 w164] -> w162
              tunnel: w151 -> [w163 w167]
              tunnel: "Select Local ADAM Channels" -> [_ w166]
              tunnel: w147 -> [_ w165]
              frame False {
              }
              frame True {
                n109 = stacked-sequence {
                  seq-local: [w168 _ _] -> [_ w178 _]
                  tunnel: w167 -> [w170 w177 _]
                  tunnel: [_ w175 _] -> w164
                  tunnel: w166 -> [w172 _ w184]
                  tunnel: w165 -> [w171 _ _]
                  frame #0 {
                    n110 = Array Size(array=w170) -> ()  [unwired: 1 out]
                    n111 = for {
                      tunnel: w170 -> [w174] mode=indexing
                      tunnel: [w173] -> w169 mode=indexing
                      n112 = Unbundle By Name(w174) -> ("Ch Name"=w173:string)
                    }
                    n113 = call "Get_local_ADAM_Chs.vi"("Local ADAM?"=w171, "Show setup"=w172, "Desired Local ADAM Channels"=w169) -> ("Choosen Channels"=w168:string[])  [unwired: 1 out]
                  }
                  frame #1 {
                    n114 = for {
                      tunnel: [w183] -> w175 mode=indexing
                      tunnel: w178 -> [w181]
                      tunnel: w177 -> [w182] mode=indexing
                      i -> [w179]
                      n115 = Index Array(array=w181, index=w179) -> (element=w180:string)
                      n116 = Bundle By Name(cluster=w182, "Ch No"=w179, "Ch Name"=w180) -> (w183:T20)
                    }
                    n117 = Array Size(array=w175) -> (size(s)=w176:i32)
                    n118 = local write "No of Analogue inst"(w176) -> ()
                  }
                  frame #2 {
                    n119 = case shown="True" w184 {
                      frame False {
                      }
                      frame True {
                        n120 = local write "Select Local ADAM Channels"(FALSE ("Select Local ADAM Channels")) -> ()
                      }
                    }
                  }
                }
              }
            }
            n121 = Select(t=w154, s=w147, f=u8 2 ("Disabled")) -> (s? t:f=w152:u8)
            n122 = property on="Ch Name" class="Str"("Visible"=w147) -> ()  [unwired: 2 in, 2 out]
            n123 = property on="Select Local ADAM Channels" class="Bool (strict)"("Disabled"=w152) -> ()  [unwired: 2 in, 2 out]
            n124 = Not(x=w147) -> (.not. x?=w146:bool)
            n125 = property on="high limit" class="DigNum (strict)"("Visible"=w146) -> ()  [unwired: 2 in, 2 out]
            n126 = property on="low limit" class="DigNum (strict)"("Visible"=w146) -> ()  [unwired: 2 in, 2 out]
            n127 = property on="Ch No" class="DigNum (strict)"("Visible"=w146) -> ()  [unwired: 2 in, 2 out]
          }
          frame #5 {
            n128 = case shown="True" "Select Plug Ins" {
              tunnel: w186 -> [_ w188]
              frame False {
              }
              frame True {
                n129 = stacked-sequence {
                  tunnel: w188 -> [w189 _]
                  frame #0 {
                    w193 = TRUE  # Show Panel?
                    n130 = global read "Meas_global.vi" "Pre Setup String"() -> (w192:string)
                    n131 = local write "Select Plug Ins"(FALSE ("Select Local ADAM Channels")) -> ()
                    n132 = call "Choose_Plug_In_to_Run.vi"("setup"=w189, "Show Panel?"=w193, "Setup String In"=w192) -> ("Setup String Out"=w191:string)  [unwired: 1 out]
                    n133 = global write "Meas_global.vi" "Pre Setup String"(w191) -> ()
                  }
                  frame #1 {
                    n134 = Current VI's Path() -> (path=w195:path)
                    n135 = call "Open_Close_Front_Panel.ph.vi"("Front Panel Window:Open"=TRUE, "VI path"=w195) -> ()  [unwired: 2 out]
                  }
                }
              }
            }
          }
          frame #6 {
            n136 = Initialize Array(0) -> (w207:i32[])  [unwired: 1 out]
            n137 = for {
              shift-right: [w214] -> w203
              shift-left: w207 -> [w215]
              tunnel: [w213] -> w201 mode=indexing
              tunnel: w200 -> [w212] mode=indexing
              tunnel: [w210] -> w199 mode=indexing
              n138 = Unbundle By Name(w212) -> ("Inst type"=w209:T2)
              n139 = case shown="\"Cross wire 1\"" w209 {
                tunnel: w215 -> [w219 w223 w225 w229]
                tunnel: [w218 w222 w225 w228] -> w214
                tunnel: [FALSE TRUE FALSE FALSE] -> w213
                frame "Propeller anemometer", Default {
                  n140 = Build Array (concatenate)(w219, 1) -> (w218:i32[])
                }
                frame "Cross wire 1" {
                  n141 = Build Array (concatenate)(w223, 2) -> (w222:i32[])
                }
                frame "Cross wire 2" {
                }
                frame "LDA Vel" {
                  n142 = Build Array (concatenate)(w229, 1) -> (w228:i32[])
                }
              }
              n143 = Equal?(x=w209, y=Inst_type."Preston tube" ("Inst type")) -> (x = y?=w210:bool)
            }
            n144 = Build Array (concatenate)(w203, 1) -> (w202:i32[])
            n145 = Array Subset(array=w202, length="No of Analogue inst") -> (w206:i32[])  [unwired: 1 in]
            n146 = Add Array Elements(numeric array=w206) -> (sum=w205:i32)
            n147 = Or Array Elements(Boolean array=w201) -> (logical OR=→"XW Present?":bool)
            n148 = Or Array Elements(Boolean array=w199) -> (logical OR=w197:bool)
            n149 = property on="D" class="DigNum (strict)"("Visible"=w197) -> ()  [unwired: 2 in, 2 out]
          }
          frame #7 {
            "Notes" <- ""
          }
          frame #8 {
            n150 = Array Size(array=w234) -> (size(s)=w233:i32)
            n151 = Not Equal To 0?(x=w233) -> (x != 0?=w232:bool)
            n152 = case shown="True" w232 {
              tunnel: [enum16{"No Analogue data", "Take Analogue data"}."No Analogue data" ("Analogue data") enum16{"No Analogue data", "Take Analogue data"}."Take Analogue data" ("Analogue data")] -> w231
              frame False {
              }
              frame True {
              }
            }
            n153 = global write "Meas_global.vi" "Analogue data"(w231) -> ()
          }
          frame #9 {
            n154 = Index Array(array=w239, index=0) -> (element=w244:T20)
            n155 = Initialize Array(w244) -> (w242:T10)  [unwired: 1 out]
            n156 = Build Array (concatenate)(w239, w244) -> (w243:T10)
            n157 = for {
              N: w240 -> [_]
              tunnel: w243 -> [w252] mode=indexing
              shift-right: [w253] -> w238
              shift-left: w242 -> [w247]
              tunnel: Inst_type."Cross wire 2" ("Inst type") -> [w245]
              shift-right: [w251] -> _
              shift-left: _ -> [w250]
              tunnel: w243 -> [w249]
              n158 = Unbundle By Name(w252) -> ("Inst type"=w251:T2)
              n159 = Array Size(array=w247) -> (size(s)=w246:i32)
              n160 = Increment(x=w246) -> (x+1=w248:i32)
              n161 = case shown="\"Cross wire 1\"" w251 {
                tunnel: [w262 w283 w295] -> w253
                tunnel: w247 -> [w263 w285 w297]
                tunnel: w252 -> [w259 w286 w296]
                tunnel: w245 -> [w261 w290 _]
                tunnel: w250 -> [_ w289 _]
                tunnel: w249 -> [w266 _ _]
                tunnel: w248 -> [w265 _ _]
                frame "Cross wire 1" {
                  n162 = Index Array(array=w266, index=w265) -> (element=w260:T20)
                  n163 = Unbundle By Name(w260) -> ("Inst type"=w264:T2, "high limit"=w257:sgl, "low limit"=w256:sgl, "Ch No"=w255:i16, "Symbol"=w254:string)
                  n164 = Unbundle By Name(w259) -> ("Calib filename"=w258:path)
                  n165 = case shown="\"Generic Linear\", Default" w264 {
                    tunnel: w263 -> [w276 w282]
                    tunnel: [w275 w281] -> w262
                    tunnel: w261 -> [w268 w277]
                    tunnel: w258 -> [w274 w280]
                    tunnel: w259 -> [w272 w278]
                    tunnel: w260 -> [_ _]
                    tunnel: w257 -> [w271 _]
                    tunnel: w256 -> [w270 _]
                    tunnel: w255 -> [w269 _]
                    tunnel: w254 -> [w267 _]
                    frame "Cross wire 2" {
                      n166 = Bundle By Name(cluster=w272, "Calib filename"=w274, "Inst type"=w268, "high limit"=w271, "low limit"=w270, "Ch No"=w269, "Symbol"=w267) -> (w273:T20)
                      n167 = Build Array (concatenate)(w276, w272, w273) -> (w275:T10)
                    }
                    frame "Generic Linear", Default {
                      n168 = Bundle By Name(cluster=w278, "Calib filename"=w280, "Inst type"=w277) -> (w279:T20)
                      n169 = Build Array (concatenate)(w282, w278, w279) -> (w281:T10)
                    }
                  }
                }
                frame "Cross wire 2" {
                  n170 = Decrement(x=w290) -> (x-1=w288:T2)
                  n171 = Equal?(x=w288, y=w289) -> (x = y?=w287:bool)
                  n172 = Bundle By Name(cluster=w286, "Inst type"=w288) -> (w284:T20)
                  n173 = case shown="False" w287 {
                    tunnel: w286 -> [_ _]
                    tunnel: w285 -> [w293 w294]
                    tunnel: w284 -> [w292 _]
                    tunnel: [w291 w294] -> w283
                    frame False {
                      n174 = Build Array (concatenate)(w293, w292) -> (w291:T10)
                    }
                    frame True {
                    }
                  }
                }
                frame "Generic Linear", Default {
                  n175 = Build Array (concatenate)(w297, w296) -> (w295:T10)
                }
              }
            }
          }
          frame #10 {
            n176 = Equal?(x=w299, y=Post_Process."Take New Data" ("Post Process")) -> (x = y?=w298:bool)
          }
          frame #11 {
            n177 = case shown="True" "OK" {
              tunnel: w301 -> [_ w318]
              tunnel: [FALSE w317] -> w303
              tunnel: w302 -> [_ w306]
              frame False {
              }
              frame True {
                n178 = for {
                  tunnel: w318 -> [w330] mode=indexing
                  tunnel: [w328] -> w312 mode=indexing
                  tunnel: [w324] -> w316 mode=indexing
                  n179 = Unbundle By Name(w330) -> ("high limit"=w333:sgl, "low limit"=w332:sgl, "Ch No"=w329:i16, "Inst type"=w327:T2, "Symbol"=w326:string)
                  n180 = Number To Decimal String(number=w327) -> (decimal integer string=w325:string)  [unwired: 1 out]
                  n181 = Concatenate Strings(w325, w326) -> (w324:string)
                  n182 = Greater Or Equal?(x=w333, y=w332) -> (x >= y?=w331:bool)
                  n183 = case shown="\"Propeller anemometer\", Default" w327 {
                    tunnel: w331 -> [w336 _ _ _]
                    tunnel: w329 -> [w335 _ _ _]
                    tunnel: [w334 TRUE TRUE TRUE] -> w328
                    frame "Propeller anemometer", Default {
                      n184 = case shown="True" w336 {
                        tunnel: w335 -> [w339 _]
                        tunnel: [FALSE TRUE] -> w334
                        frame False {
                          n185 = Number To Decimal String(number=w339) -> (decimal integer string=w338:string)  [unwired: 1 out]
                          n186 = Concatenate Strings("Error in input limits for Channel No ", w338) -> (w340:string)
                          n187 = One Button Dialog(message=w340) -> ()  [unwired: 2 out]
                        }
                        frame True {
                        }
                      }
                    }
                    frame "LDA Vel" {
                    }
                    frame "LDA Tran time" {
                    }
                    frame "LDA Arr time" {
                    }
                  }
                }
                n188 = call "Analyse_string_array.vi"("String array"=w316) -> ("Frequency"=w315:i32[])  [unwired: 2 out]
                n189 = global read "Meas_global.vi" "Remote control"() -> (w307:bool)
                n190 = Greater?(x=w315, y=1) -> (0:w313:bool[])
                n191 = Or Array Elements(Boolean array=w313) -> (logical OR=w309:bool)
                n192 = Compound Arithmetic op=AND(invert w307, w309, w306) -> (w308:bool)
                n193 = case shown="True" w308 {
                  tunnel: [TRUE FALSE] -> w311
                  frame False {
                  }
                  frame True {
                    n194 = Current VI's Path() -> (path=w321:path)
                    n195 = call "Open_Close_Front_Panel.ph.vi"("Front Panel Window:Open"=TRUE, "VI path"=w321) -> ()  [unwired: 2 out]
                    n196 = One Button Dialog(message="Non Unique symbol names") -> ()  [unwired: 2 out]
                  }
                }
                n197 = Build Array (concatenate)(w312, w311) -> (w310:bool[])
                n198 = And Array Elements(Boolean array=w310) -> (logical AND=w317:bool)
              }
            }
          }
          frame #12 {
            n199 = And(x=w349, y=w348) -> (x .and. y?=w351:bool)
            n200 = case shown="True" w351 {
              tunnel: w346 -> [_ w359]
              tunnel: [FALSE w358] -> w352
              tunnel: [w353 w357] -> w350
              tunnel: w348 -> [w354 _]
              tunnel: w347 -> [_ _]
              frame False {
                n201 = Not(x=w354) -> (.not. x?=w353:bool)
              }
              frame True {
                n202 = for {
                  shift-right: [w378] -> _
                  shift-left: i16[] [] -> [w377]
                  tunnel: w359 -> [w374] mode=indexing
                  tunnel: [w365] -> w360 mode=indexing
                  shift-right: [w373] -> _
                  shift-left: path[] [] -> [w372]
                  n203 = Unbundle By Name(w374) -> ("Ch No"=w375:i16)
                  n204 = Unbundle By Name(w374) -> ("Inst type"=w371:T2, "Calib filename"=w368:path)
                  n205 = Search 1D Array(1D array=w377, element=w375) -> (index of element=w376:i32)  [unwired: 1 out]
                  n206 = Build Array (concatenate)(w377, w375) -> (w378:i16[])
                  n207 = Equal?(x=Inst_type."Fast FID" ("Inst type"), y=w371) -> (x = y?=w364:bool)
                  n208 = case shown="0, Default" w376 {
                    tunnel: w375 -> [w389 _]
                    tunnel: [w385 FALSE ("true")] -> w367
                    frame 0, Default {
                      n209 = Format Into String(format string="The Ch No %d appears more than once", w389) -> (resulting string=w387:string)  [unwired: 2 in, 1 out]
                      n210 = One Button Dialog(message=w387, button name ("OK")="Ok") -> (true=w385:bool)
                    }
                    frame -1 {
                    }
                  }
                  n211 = Search 1D Array(1D array=w372, element=w368) -> (index of element=w369:i32)  [unwired: 1 out]
                  n212 = Greater Or Equal To 0?(x=w369) -> (x >= 0?=w363:bool)
                  n213 = And(x=w364, y=w363) -> (x .and. y?=w362:bool)
                  n214 = case shown="True" w362 {
                    tunnel: [w380 FALSE ("true")] -> w366
                    tunnel: w368 -> [w379 _]
                    frame True {
                      n215 = Format Into String(format string="Calibration file %s is used more than once.", w379) -> (resulting string=w382:string)  [unwired: 2 in, 1 out]
                      n216 = One Button Dialog(message=w382, button name ("OK")="Ok") -> (true=w380:bool)
                    }
                    frame False {
                    }
                  }
                  n217 = Build Array (concatenate)(w372, w368) -> (w373:path[])
                  n218 = Or(x=w367, y=w366) -> (x .or. y?=w365:bool)
                }
                n219 = Or Array Elements(Boolean array=w360) -> (logical OR=w357:bool)
                n220 = Not(x=w357) -> (.not. x?=w358:bool)
              }
            }
          }
          frame #13 {
            n221 = call "Current_Calib_Filenames.vi"("Mode"=App_Global."Read Global") -> ("Calib Filename Out"=w392:path[], "Channel Numbers Out"=w393:i16[])  [unwired: 2 in, 1 out]
            n222 = for {
              tunnel: w391 -> [w406] mode=indexing
              tunnel: w393 -> [w408]
              tunnel: w392 -> [w407]
              tunnel: [w405] -> w395 mode=indexing
              w403 = Inst_type."Cross wire 2"  # Inst type
              n223 = Unbundle By Name(w406) -> ("Inst type"=w398:T2, "Ch No"=w400:i16, "Use Latest"=w401:bool, "Inst type"=w404:T2)
              n224 = Not Equal?(x=w404, y=w403) -> (x != y?=w402:bool)
              n225 = Compound Arithmetic op=AND(w401, w402) -> (w399:bool)
              n226 = Not Equal?(x=Inst_type."Raw voltage" ("Inst type"), y=w398) -> (x != y?=w396:bool)
              n227 = case shown="True" w399 {
                tunnel: w408 -> [_ w419]
                tunnel: w400 -> [_ w418]
                tunnel: w407 -> [_ w416]
                tunnel: w406 -> [w409 w415]
                tunnel: [w409 w414] -> w405
                tunnel: w396 -> [_ w411]
                frame False {
                }
                frame True {
                  n228 = Search 1D Array(1D array=w419, element=w418) -> (index of element=w417:i32)  [unwired: 1 out]
                  n229 = Index Array(array=w416, index=w417) -> (element=w412:path)
                  n230 = Select(t=w412, s=w411, f=path "") -> (s? t:f=w413:path)
                  n231 = Bundle By Name(cluster=w415, "Calib filename"=w413) -> (w414:T20)
                }
              }
            }
          }
          frame #14 {
            n232 = case shown="True" w421 {
              tunnel: w420 -> [w425 w428]
              tunnel: [w425 w427] -> w424
              tunnel: w423 -> [_ _]
              tunnel: w422 -> [_ w426]
              frame False {
              }
              frame True {
                n233 = case shown="\"Run Program\", Default" w426 {
                  tunnel: w428 -> [w430 w438]
                  tunnel: [w429 w438] -> w427
                  frame "Run Program", Default {
                    n234 = for {
                      tunnel: w430 -> [w431] mode=indexing
                      tunnel: [w432] -> w429 mode=indexing
                      n235 = Unbundle By Name(w431) -> ("Calib filename"=w437:path, "Use Latest"=w436:bool, "Ch No"=w435:i16, "Inst type"=w434:T2)
                      n236 = call "Find_calibration_file.vi"("Inst type"=w434, "Ch No"=w435, "Use Latest Calib"=w436, "filename"=w437) -> ("filename out"=w433:path)
                      n237 = Bundle By Name(cluster=w431, "Calib filename"=w433) -> (w432:T20)
                    }
                  }
                  frame "Setup Front Panel" {
                  }
                }
              }
            }
          }
          frame #15 {
            w441 = 0 ("Index")
            n238 = Index Array(array=w443, index=w441) -> (element=w442:T20)
            n239 = Initialize Array(w442, w441) -> (w440:T10)
            n240 = for {
              shift-right: [w451] -> w445
              shift-left: w440 -> [w450]
              shift-right: [w452] -> w446
              shift-left: w440 -> [w454]
              tunnel: w443 -> [w453] mode=indexing
              n241 = Unbundle By Name(w453) -> ("Move channel"=w455:bool)
              n242 = case shown="True" w455 {
                tunnel: w454 -> [w457 w463]
                tunnel: w453 -> [w459 w462]
                tunnel: [w458 w463] -> w452
                tunnel: [w456 w461] -> w451
                tunnel: w450 -> [w456 w460]
                frame False {
                  n243 = Build Array (concatenate)(w457, w459) -> (w458:T10)
                }
                frame True {
                  n244 = Build Array (concatenate)(w460, w462) -> (w461:T10)
                }
              }
            }
            n245 = Build Array (concatenate)(w446, w445) -> (w444:T10)
            n246 = for {
              tunnel: w444 -> [w449] mode=indexing
              tunnel: [w447] -> w439 mode=indexing
              n247 = Bundle By Name(cluster=w449, "Move channel"=FALSE) -> (w447:T20)
            }
          }
          frame #16 {
            n248 = for {
              shift-right: [w473] -> _
              shift-left: string[] [] -> [w474]
              tunnel: [w476] -> w465 mode=indexing
              tunnel: [w470] -> w466 mode=indexing
              tunnel: w467 -> [w472] mode=indexing
              tunnel: [w469] -> w464 mode=indexing
              n249 = Unbundle By Name(w472) -> ("Inst type"=w475:T2)
              n250 = case shown="\"Propeller anemometer\"" w475 {
                tunnel: [w483 w487 w490 w494 w498 w502 w506 "XW" w513 w518 w521 w525] -> w470
                tunnel: ["U" "P" "U" "U" "tau" "U" "U" "W" "U" "C" "T" "T"] -> w477
                tunnel: w474 -> [w484 w488 w492 w496 w500 w504 w508 w510 w515 w519 w523 w527]
                tunnel: [w482 w486 w491 w495 w499 w503 w507 w510 w514 w517 w522 w526] -> w473
                frame "Propeller anemometer" {
                  w483 = "Prop"
                  n251 = Build Array (concatenate)(w484, w483) -> (w482:string[])
                }
                frame "Pressure Transducer" {
                  w487 = "Mano"
                  n252 = Build Array (concatenate)(w488, w487) -> (w486:string[])
                }
                frame "Raw voltage" {
                  w490 = "RV"
                  n253 = Build Array (concatenate)(w492, w490) -> (w491:string[])
                }
                frame "Pitot-static tube" {
                  w494 = "Pitot"
                  n254 = Build Array (concatenate)(w496, w494) -> (w495:string[])
                }
                frame "Preston tube" {
                  w498 = "Preston"
                  n255 = Build Array (concatenate)(w500, w498) -> (w499:string[])
                }
                frame "Hot wire" {
                  w502 = "HW"
                  n256 = Build Array (concatenate)(w504, w502) -> (w503:string[])
                }
                frame "Cross wire 1" {
                  w506 = "XW"
                  n257 = Build Array (concatenate)(w508, w506) -> (w507:string[])
                }
                frame "Cross wire 2" {
                }
                frame "Generic Linear", Default {
                  w513 = "Gen"
                  n258 = Build Array (concatenate)(w515, w513) -> (w514:string[])
                }
                frame "Fast FID" {
                  w518 = "FF"
                  n259 = Build Array (concatenate)(w519, w518) -> (w517:string[])
                }
                frame "Thermocouple" {
                  w521 = "T"
                  n260 = Build Array (concatenate)(w523, w521) -> (w522:string[])
                }
                frame "Cold wire" {
                  w525 = "CW"
                  n261 = Build Array (concatenate)(w527, w525) -> (w526:string[])
                }
              }
              n262 = call "Analyse_string_array.vi"("String array"=w473) -> ("Unique strings"=w481:string[], "Frequency"=w479:i32[])  [unwired: 1 out]
              n263 = Search 1D Array(1D array=w481, element=w470) -> (index of element=w480:i32)  [unwired: 1 out]
              n264 = Index Array(array=w479, index=w480) -> (element=w471:i32)
              n265 = Number To Decimal String(number=w471) -> (decimal integer string=w469:string)  [unwired: 1 out]
              n266 = Concatenate Strings(w469, w470, ":", w477) -> (w476:string)
            }
          }
          frame #17 {
            w539 = T8 {"Colour"=0, "Inst type"=enum."Pitot-static tube", "Inst name"="Manometer voltage", "Symbol"="U", "Code name"="", "Extra Info"="U", "Inst Array"=enum."PWA", "Extra Titles"=[], "Extra Values"=[], "U"=0.0, "u^2"=0.0, "u^3"=0.0, "u^4"=0.0, "Skew_u"=0.0, "Kurt_u"=0.0, "Sd Error in Mean"=0.0, "% u'/U"=0.0, "X"=0.0, "Y"=0.0, "Z"=0.0, "Timescale integral to 25%"=0.0, "Sd Error in Variance"=0.0, "Calib File"=path "", "Calib Constants"=[], "Output Position"=FALSE, "Full Stats"=FALSE, "Av Sampling Rate"=0.0, "Av No of Samples"=0.0, "Total Meas Time (s)"=0.0, "ADAM Ch Name"=""}  # Analysis info cluster
            n267 = property on="Ch Name" class="Str"() -> ("Visible"=w540:bool)  [unwired: 2 in, 2 out]
            n268 = global read "Meas_global.vi" "Pre Setup String"() -> (w531:string)
            n269 = for {
              tunnel: [w571] -> w538 mode=indexing
              tunnel: w533 -> [w547] mode=indexing
              tunnel: w536 -> [w562] mode=indexing
              tunnel: T14 {"high limit (10V)"=10.0, "low limit (-10V)"=-10.0, "Ch No"=0, "Var name"="", "Use Latest Calib"=FALSE} ("Ch and Spans") -> [w568]
              tunnel: [w567] -> w532 mode=indexing
              tunnel: w535 -> [w550] mode=indexing
              tunnel: w539 -> [w565]
              tunnel: w534 -> [w559] mode=indexing
              tunnel: w540 -> [w542]
              tunnel: w531 -> [w551]
              tunnel: [w546] -> w530 mode=indexing
              tunnel: w529 -> [w541]
              n270 = Unbundle By Name(w547) -> ("Use Latest"=w563:bool, "high limit"=w570:sgl, "low limit"=w569:sgl, "Ch No"=w564:i16, "Inst type"=w557:T2, "Symbol"=w556:string, "D"=w555:dbl, "Ch Name"=w543:string)
              n271 = Empty String/Path?(string/path=w556) -> (empty?=w560:bool)
              n272 = Concatenate Strings(w550, "_ADAM_Ch_Name" ("string")) -> (w548:string)
              n273 = call "Get_Characters_from_string.vi"("Input string"=w551, "Variable name"=w548) -> ("Value"=w545:string)  [unwired: 1 in, 1 out]
              n274 = Select(t=w559, s=w560, f=w556) -> (s? t:f=w558:string)
              n275 = Format Into String(format string="%s (%s)" ("Format String"), w562, w558) -> (resulting string=w553:string)  [unwired: 2 in, 1 out]
              n276 = Select(t=w543, s=w542, f=w553) -> (s? t:f=w552:string)
              n277 = Bundle By Name(cluster=w568, "Use Latest Calib"=w563, "high limit (10V)"=w570, "low limit (-10V)"=w569, "Ch No"=w564, "Var name"=w552) -> (w571:T14)
              n278 = Select(t=w545, s=w541, f=w543) -> (s? t:f=w544:string)
              n279 = case shown="\"Propeller anemometer\", Default" w557 {
                tunnel: [w574 w577] -> w566
                tunnel: w564 -> [w572 _]
                tunnel: w555 -> [_ w575]
                frame "Propeller anemometer", Default {
                  n280 = Format Into String(format string="Ch %d" ("Format String"), w572) -> (resulting string=w574:string)  [unwired: 2 in, 1 out]
                }
                frame "Preston tube" {
                  n281 = Format Into String(format string="D = %.2f" ("Format String"), w575) -> (resulting string=w577:string)  [unwired: 2 in, 1 out]
                }
              }
              n282 = Bundle By Name(cluster=w547, "Ch Name"=w544) -> (w546:T20)
              n283 = Bundle By Name(cluster=w565, "Extra Info"=w566, "Inst type"=w557, "Inst name"=w553, "Symbol"=w558, "Code name"=w550, "Inst Array"=Instrument_Array."Analogue", "ADAM Ch Name"=w544) -> (w567:T8)
            }
            n284 = global write "Meas_global.vi" "Ch & spans"(w538) -> ()
          }
          frame #18 {
            n285 = Not Equal?(x=w579, y=w578) -> (x != y?=w580:bool)
            n286 = case shown="True" w580 {
              tunnel: w578 -> [_ w581]
              frame False {
              }
              frame True {
                n287 = local write "Ch & spans choices"(w581) -> ()
              }
            }
          }
          frame #19 {
            n288 = global read "Meas_global.vi" "Duplicate channels"() -> (w583:i32[])
            n289 = case shown="True" "Select Duplicate Channels" {
              tunnel: w586 -> [_ _]
              tunnel: w584 -> [w594 w617]
              tunnel: w583 -> [w588 w610]
              tunnel: [w587 w609] -> w582
              frame False {
                n290 = for {
                  tunnel: w594 -> [w608] mode=indexing
                  tunnel: [w607] -> w595 mode=indexing
                  n291 = Unbundle By Name(w608) -> ("Inst type"=w607:T2)
                }
                n292 = for {
                  tunnel: w588 -> [w604] mode=indexing
                  tunnel: w595 -> [w606]
                  tunnel: [w605] -> w599 mode=indexing
                  tunnel: [w604] -> w596 mode=indexing
                  n293 = Index Array(array=w606, index=w604) -> (element=w605:T2)
                }
                n294 = Array Size(array=w594) -> (size(s)=w597:i32)
                n295 = Array Max & Min(array=w599) -> (max value=w600:T2, min value=w601:T2)  [unwired: 2 out]
                n296 = Array Max & Min(array=w596) -> (max index (indices)=w598:i32)  [unwired: 3 out]
                n297 = Array Size(array=w588) -> (size(s)=w593:i32)
                n298 = Equal?(x=w600, y=w601) -> (x = y?=w603:bool)
                n299 = Greater?(x=w593, y=1) -> (0:w590:bool)
                n300 = Greater?(x=w597, y=w598) -> (0:w602:bool)
                n301 = Compound Arithmetic op=AND(w590, w603, w602) -> (w589:bool)
                n302 = Select(t=w588, s=w589, f=i32[] [] ("32bit integer")) -> (s? t:f=w587:i32[])
              }
              frame True {
                n303 = for {
                  tunnel: w617 -> [w624] mode=indexing
                  shift-right: [w619] -> w613
                  shift-left: string[] [] -> [w620]
                  tunnel: w610 -> [w622]
                  tunnel: [w618] -> w612 mode=indexing
                  i -> [w623]
                  n304 = Unbundle By Name(w624) -> ("Inst name"=w618:string)
                  n305 = Search 1D Array(1D array=w622, element=w623) -> (index of element=w621:i32)  [unwired: 1 out]
                  n306 = case shown="0, Default" w621 {
                    tunnel: w620 -> [w627 w628]
                    tunnel: w618 -> [w626 _]
                    tunnel: [w625 w628] -> w619
                    frame 0, Default {
                      n307 = Build Array (concatenate)(w627, w626) -> (w625:string[])
                    }
                    frame -1 {
                    }
                  }
                }
                n308 = call "Select_Strings.vi"("Available Ch names"=w612, "Message"="Please select similar instruments whose results columns will be combined", "Selector mode"=T15."Zero or more", "Desired Ch names (in)"=w613) -> ("Ch Indicies Choosen"=w609:i32[])  [unwired: 4 out]
                n309 = local write "Select Duplicate Channels"(FALSE ("Select Local ADAM Channels")) -> ()
              }
            }
            n310 = global write "Meas_global.vi" "Duplicate channels"(w582) -> ()
          }
          frame #20 {
            n311 = local read "XW Present?"() -> (w631:bool)
            n312 = property on="Cross wire/LDA" class="Enum (strict)"("Visible"=w631) -> ()  [unwired: 2 in, 2 out]
            n313 = case shown="\"Take LDA data\"" "LDA data" {
              tunnel: [w640 w643] -> w633
              tunnel: w634 -> [_ w641]
              tunnel: w635 -> [_ _]
              tunnel: [w640 w642] -> w630
              frame "No LDA data" {
                w639 = FALSE  # Synchronise Analogue channels with LDA
                w640 = u8 2  # Disabled
                n314 = local write "Synchronise Analogue channels with LDA"(w639) -> ()
              }
              frame "Take LDA data" {
                n315 = stacked-sequence {
                  tunnel: [w644 _] -> w643
                  tunnel: [_ w646] -> w642
                  tunnel: w641 -> [_ w647]
                  frame #0 {
                    w644 = u8 0  # Disabled
                  }
                  frame #1 {
                    n316 = Array Size(array=w647) -> (size(s)=w648:i32)
                    n317 = Not Equal To 0?(x=w648) -> (x != 0?=w645:bool)
                    n318 = case shown="False" w645 {
                      tunnel: w645 -> [w650 _]
                      tunnel: [w649 w651] -> w646
                      frame False {
                        w649 = u8 2  # Disabled
                        n319 = local write "Synchronise Analogue channels with LDA"(w650) -> ()
                      }
                      frame True {
                        w651 = u8 0  # Disabled
                      }
                    }
                  }
                }
              }
            }
            n320 = case shown="True" w631 {
              tunnel: [w637 "Cross wire"] -> w629
              frame False {
                w637 = T7."2nd component as calculated"  # Cross wire/LDA
              }
              frame True {
              }
            }
            n321 = global write "Meas_global.vi" "Cross wire + or -ve"(w629) -> ()
            n322 = Wait (ms)(milliseconds to wait=u32 100) -> ()  [unwired: 1 out]
            n323 = property on="Synchronise Analogue channels with LDA" class="Bool (strict)"("Disabled"=w630) -> ()  [unwired: 2 in, 2 out]
            n324 = property on="LDA set up" class="Clust (strict)"("Disabled"=w633) -> ()  [unwired: 2 in, 2 out]
          }
          frame #21 {
            n325 = And(x=w657, y=w658) -> (x .and. y?=w656:bool)
            n326 = local read "Synchronise Analogue channels with LDA"() -> (w655:bool)
            n327 = while {
              shift-left: _ -> [w684]
              shift-right: [w685] -> w652
              tunnel: [w686] -> w654
              stop <- FALSE continue-if-true
              n328 = local read "Setup filename selector"() -> (w685:u16)
              n329 = Not Equal?(x=w685, y=w684) -> (x != y?=w686:bool)
            }
            n330 = case shown="True" w655 {
              tunnel: w659 -> [_ w670]
              tunnel: w656 -> [_ w669]
              frame False {
              }
              frame True {
                n331 = case shown="True" w669 {
                  tunnel: w670 -> [_ w673]
                  frame False {
                  }
                  frame True {
                    n332 = for {
                      tunnel: w673 -> [w682] mode=indexing
                      tunnel: [w675] -> w672 mode=indexing
                      n333 = Unbundle By Name(w682) -> ("Inst type"=w681:T2, "Symbol"=w679:string)
                      n334 = Equal?(x=w679, y="Sync") -> (x = y?=w677:bool)
                      n335 = Equal?(x=Inst_type."Raw voltage" ("Inst type"), y=w681) -> (x = y?=w676:bool)
                      n336 = And(x=w676, y=w677) -> (x .and. y?=w675:bool)
                    }
                    n337 = Or Array Elements(Boolean array=w672) -> (logical OR=w671:bool)
                    n338 = case shown="False" w671 {
                      frame False {
                        n339 = One Button Dialog(message="To Perform LDA Sync you must provide a Raw voltage channel having the symbol \"Sync\"") -> ()  [unwired: 2 out]
                      }
                      frame True {
                      }
                    }
                  }
                }
              }
            }
            n340 = case shown="True" w654 {
              tunnel: [FALSE ("exists?") w668] -> w653
              tunnel: w652 -> [_ w666]
              frame False {
              }
              frame True {
                n341 = local read "Setup Paths"() -> (w667:string[])
                n342 = Index Array(array=w667, index=w666) -> (element=w664:string)
                n343 = call "Setup_Filepath.vi"("Setup File Type"=Setup_Filetype."Measurement Setups", "Filename in"=w664) -> ("Filename Out"=w663:path)  [unwired: 1 out]
                n344 = call "Does_file_exist_(simple).vi"("Pathname"=w663) -> ("exists?"=w668:bool)
              }
            }
            n345 = local write "Read Setup File?"(w653) -> ()
            n346 = Current VI's Path() -> (path=w660:path)
            n347 = call "Close_Panel_and_Abort.vi"("Vi path"=w660, "stop"="stop") -> ()  [unwired: 1 out]
          }
        }
      }
    }
    frame #5 {
      n348 = local read "LDA data"() -> (w689:enum16{"No LDA data", "Take LDA data"})
      n349 = case shown="\"Take LDA data\"" w689 {
        tunnel: [FALSE ("Synchronise Analogue channels with LDA") "Synchronise Analogue channels with LDA"] -> w688
        frame "No LDA data" {
        }
        frame "Take LDA data" {
        }
      }
      n350 = global write "Meas_global.vi" "Synchronise with LDA"(w688) -> ()
      n351 = global write "Meas_global.vi" "LDA data"(w689) -> ()
      n352 = global write "Meas_global.vi" "LDA set up"("LDA set up") -> ()
    }
    frame #6 {
      n353 = stacked-sequence {
        seq-local: [_ w729 _ _] -> [_ _ _ w787]
        seq-local: [_ _ w755 _] -> [_ _ _ w786]
        seq-local: [w697 _ _ _] -> [_ _ _ w774]
        tunnel: w694 -> [w696 _ _ w778]
        tunnel: w693 -> [_ _ _ w777]
        tunnel: w692 -> [w695 _ _ _]
        frame #0 {
          n354 = local read "PWA Data"() -> (w698:T1)
          n355 = case shown="\"One Ch PWA\"" w698 {
            tunnel: ["" w707] -> w697
            tunnel: w696 -> [_ w706]
            tunnel: w695 -> [_ w702]
            frame "No PWA Data" {
            }
            frame "One Ch PWA" {
              n356 = Not Equal?(x="Calib_Setup.xls", y=w702) -> (x != y?=w701:bool)
              n357 = case shown="\"Setup Front Panel\"" w706 {
                tunnel: [w711 w714 w717 w720] -> w705
                tunnel: [w710 w713 w716 w719] -> w704
                tunnel: [w709 w712 w715 w718] -> w700
                tunnel: w701 -> [w709 w712 w715 _]
                frame "Show Setup" {
                  w711 = TRUE  # Show Panel?
                  w710 = T4 FALSE  # OK
                }
                frame "Run Program" {
                  w714 = FALSE  # Show Panel?
                  w713 = T4 TRUE  # OK
                }
                frame "Save Current Setup" {
                  w717 = FALSE  # Show Panel?
                  w716 = T4 TRUE  # OK
                }
                frame "Setup Front Panel" {
                  w718 = FALSE  # Check Calib file?
                  w720 = FALSE  # Show Panel?
                  w719 = T4 TRUE  # OK
                }
              }
              n358 = global read "Meas_global.vi" "Pre Setup String"() -> (w708:string)
              n359 = call "PWA_Setup_Panel.vi"("Show Panel?"=w705, "Check Calib file?"=w700, "OK"=w704, "Incoming Setup String"=w708) -> ("Outgoing Setup String"=w707:string)  [unwired: 3 out]
            }
          }
        }
        frame #1 {
          n360 = local read "LDA set up"() -> (w734:T6)
          n361 = global read "Meas_global.vi" "Duplicate channels"() -> (w733:i32[])
          n362 = Unbundle By Name(w734) -> ("dimensions"=w726:enum16{"1D", "2D"}, "Analogue Freq Multiplier"=w724:dbl)
          n363 = case shown="\"2D\"" w726 {
            tunnel: ["1D" "2D"] -> w728
            frame "1D" {
            }
            frame "2D" {
            }
          }
          n364 = for {
            shift-right: [w737] -> w731
            shift-left: "" -> [w740]
            tunnel: w733 -> [w741] mode=indexing
            n365 = Number To Decimal String(number=w741) -> (decimal integer string=w739:string)  [unwired: 1 out]
            n366 = Concatenate Strings(w740, w739, "; ") -> (w737:string)
          }
          n367 = call "Characters_to_string.vi"("Characters to write"=w728, "Label for characters"="LDA Dimensions") -> ("Output string"=w727:string)
          n368 = call "Value_to_string.vi"("Value"=w724, "Label for value"="LDA Analog Freq Multiplier") -> ("Output string"=w721:string)  [unwired: 1 in]
          n369 = call "Characters_to_string.vi"("Characters to write"=w731, "Label for characters"="Log_Similar_Measurements_in_the _same_column") -> ("Output string"=w722:string)
          n370 = Concatenate Strings(w727, w721, w722) -> (w729:string)
        }
        frame #2 {
          n371 = global write "Meas_global.vi" "Trigger mode"("Trigger mode") -> ()
          n372 = local read "Cross wire"() -> (w758:T7)
          n373 = global read "Preference_global.vi" "Rig Setup"() -> (w744:string)
          n374 = Match Pattern(string=w744, regular expression="-") -> (before substring=w743:string)  [unwired: 4 out]
          n375 = case shown="\"Free Running\"" "Trigger mode" {
            tunnel: ["Free Running" "Trigger Every Block" "Trigger Every Sample" "Start on Trigger"] -> w753
            frame "Free Running" {
            }
            frame "Trigger Every Block" {
            }
            frame "Trigger Every Sample" {
            }
            frame "Start on Trigger" {
            }
          }
          n376 = property on="PWA Data" class="Enum (strict)"() -> ("Strings []"=w749:string[])  [unwired: 2 in, 2 out]
          n377 = global write "Meas_global.vi" "PWA Data"("PWA Data") -> ()
          n378 = Equal?(x=T7."2nd component multipled by -1" ("Cross wire/LDA"), y=w758) -> (x = y?=w757:bool)
          n379 = case shown="\"EnFlo_Tunnel\"" w743 {
            tunnel: ["" w765] -> w742
            frame "False", Default {
            }
            frame "EnFlo_Tunnel" {
              n380 = call "Characters_to_string.vi"("Characters to write"="FALSE", "Label for characters"="Show_all_EnFlo_Tunnel_Columns") -> ("Output string"=w765:string)
            }
          }
          n381 = Index Array(array=w749, index="PWA Data") -> (element=w748:string)
          n382 = Select(t="TRUE", s=w757, f="FALSE") -> (s? t:f=w760:string)
          n383 = call "Characters_to_string.vi"("Characters to write"=w748, "Label for characters"="Pulsed_Wire_Data" ("Variable name")) -> ("Output string"=w747:string)
          n384 = call "Characters_to_string.vi"("Characters to write"=w760, "Label for characters"="Invert Second Component") -> ("Output string"=w756:string)
          n385 = call "Characters_to_string.vi"("Characters to write"=w753, "Label for characters"="Trigger mode") -> ("Output string"=w751:string)
          n386 = Concatenate Strings(w751, w747, w756, w742) -> (w755:string)
        }
        frame #3 {
          w779 = FALSE  # Show Panel?
          n387 = for {
            tunnel: w777 -> [w792] mode=indexing
            tunnel: [w791] -> w773 mode=indexing
            n388 = Unbundle By Name(w792) -> ("Ch Name"=w791:string)
          }
          n389 = global read "Meas_global.vi" "Pre Setup String"() -> (w780:string)
          n390 = call "Choose_Plug_In_to_Run.vi"("setup"=w778, "Show Panel?"=w779, "Setup String In"=w780) -> ("Setup String Out"=w781:string)  [unwired: 1 out]
          n391 = Array To Spreadsheet String(array=w773, 3:"%s" ("format string")) -> (spreadsheet string=w775:string)  [unwired: 1 out]
          n392 = call "Add_label_to_string.vi"("String to write"=w775, "File Label"="Local ADAM Channels") -> ("Output string"=w788:string)
          n393 = call "Date_and_Time_to_string.vi"() -> ("Date and time (spreadsheet)"=w783:string)
          n394 = global read "Meas_global.vi" "New Setup String"() -> (w782:string)
          n395 = call "Value_to_string.vi"("Value"="Sync Delay Time (ms)", "Label for value"="Sync Delay Time (ms)" ("Label for characters")) -> ("Output string"=w776:string)  [unwired: 1 in]
          n396 = Concatenate Strings(w782, w774, w781, w783, w787, w786, w788, w776) -> (w790:string)
          n397 = global write "Meas_global.vi" "New Setup String"(w790) -> ()
          n398 = global write "LDA_meas_global_1.vi" "Sync Delay Time (ms)"("Sync Delay Time (ms)") -> ()
        }
      }
    }
    frame #7 {
      n399 = case shown="\"Post Process Raw Data File\"" w795 {
        tunnel: w794 -> [w802 w837]
        tunnel: [w796 w831] -> w793
        frame "Take New Data" {
          n400 = for {
            tunnel: w802 -> [w813] mode=indexing
            shift-right: [w809] -> w799
            shift-left: i16[] [] -> [w811]
            shift-right: [w807] -> w798
            shift-left: path[] [] -> [w808]
            tunnel: [w804] -> w796 mode=indexing
            n401 = Unbundle By Name(w813) -> ("Use Latest"=w806:bool, "Inst type"=w812:T2, "Ch No"=w810:i16, "Calib filename"=w805:path)
            n402 = call "Current_Filepath.vi"("Filename in"=w805, "Data Type"="Calibrations") -> ("Filename Out"=w804:path)  [unwired: 1 out]
            n403 = case shown="\"Propeller anemometer\", Default" w812 {
              tunnel: w811 -> [w820 w830]
              tunnel: w810 -> [w819 _]
              tunnel: [w818 w830] -> w809
              tunnel: w808 -> [w817 w829]
              tunnel: w805 -> [w816 _]
              tunnel: [w815 w829] -> w807
              tunnel: w806 -> [w814 _]
              frame "Propeller anemometer", Default {
                n404 = case shown="False" w814 {
                  tunnel: w820 -> [w826 w828]
                  tunnel: w819 -> [w825 _]
                  tunnel: [w824 w828] -> w818
                  tunnel: w817 -> [w823 w827]
                  tunnel: w816 -> [w822 _]
                  tunnel: [w821 w827] -> w815
                  frame False {
                    n405 = Build Array (concatenate)(w826, w825) -> (w824:i16[])
                    n406 = Build Array (concatenate)(w823, w822) -> (w821:path[])
                  }
                  frame True {
                  }
                }
              }
              frame "Raw voltage" {
              }
            }
          }
          n407 = call "Current_Calib_Filenames.vi"("Calib Filename"=w798, "Channel Numbers"=w799, "Mode"=App_Global."Write to Global") -> ()  [unwired: 3 out]
        }
        frame "Post Process Raw Data File" {
          n408 = for {
            tunnel: w837 -> [w843] mode=indexing
            tunnel: [w842] -> w831 mode=indexing
            n409 = Unbundle By Name(w843) -> ("Calib filename"=w842:path)
          }
          n410 = global read "Meas_global.vi" "Pre Setup String"() -> (w836:string)
          n411 = call "Get_Characters_from_string.vi"("Input string"=w836, "Variable name"="Skip_Block_Numbers_(eg 1;2;5;12)") -> ("Status"=w834:enum16{"Char in string", "Char not in string"}, "Value"=w833:string)  [unwired: 1 in]
          n412 = case shown="\"Char in string\"" w834 {
            tunnel: w833 -> [w840 _]
            tunnel: [w838 i32[] []] -> w832
            frame "Char in string" {
              n413 = call "Get_array_values_fr_String.vi"("String Value"=w840) -> ("Numeric Array"=w839:dbl[])  [unwired: 1 out]
              n414 = To Long Integer(number=w839) -> (32bit integer=w838:i32[])
            }
            frame "Char not in string" {
            }
          }
          n415 = global write "Meas_global.vi" "Blocks to Skip"(w832) -> ()
        }
      }
    }
    frame #8 {
      n416 = global read "Meas_global.vi" "Pre Setup String"() -> (w844:string)
      n417 = for {
        tunnel: [w855] -> w847 mode=indexing
        tunnel: w846 -> [w852] mode=indexing
        tunnel: w845 -> [w854] mode=indexing
        tunnel: w844 -> [w853]
        n418 = Unbundle By Name(w852) -> ("Code name"=w851:string)
        n419 = Concatenate Strings(w851, "_Av_SamplingRate" ("string")) -> (w849:string)
        n420 = call "Get_value_from_string.vi"("Input string"=w853, "Variable name"=w849) -> ("Value"=w848:dbl)  [unwired: 1 in, 1 out]
        n421 = Bundle By Name(cluster=w852, "Calib File"=w854, "Av Sampling Rate"=w848) -> (w855:T8)
      }
      "Analysis Info cluster" <- w847
    }
  }
